vi "TDMS_set-motor-test.vi"() -> ()   [LabVIEW 2015]
uses:
  TDMS_use_state.ctl
  <vilib>/Platform/TimedLoop/XDataNode/timing_clust.ctl
  <vilib>/Platform/TimedLoop/XDataNode/nitl_modes.ctl
  <vilib>/Platform/TimedLoop/XDataNode/wakeup.ctl
  <vilib>/Rock Robotics/WPI/Utilities/WPI_GetSetVariantRefNum.vi
  <vilib>/platform/TimedLoop/XDataNode/XDataNode.xnode
  <vilib>/Platform/TimedLoop/XDataNode/XDNodeRunTimeDep.lvlib
panel:
  out "x != 0?":bool
  in  "New file?":bool
  in  "Run":bool
  in  "Start logging":bool
  in  "stop logging":bool
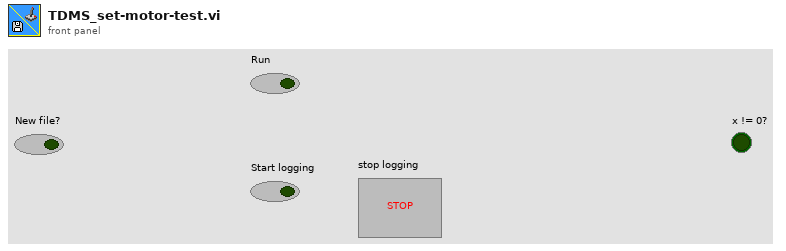
[diagram p1: front panel]
types:
  T1 = enum16{"open", "open or create", "create or replace", "create", "open (read-only)"}
  T2 = typedef "TDMS_use_state.ctl" = enum16{"Log", "Use", "Idle"}
  T3 = typedef "WPI_MotorControlDeviceRef.ctl" = cluster{"DeviceStatus":errorcluster, "Type":T4, "PWM":cluster{"PWM Channel":T5, "DeadBand":T6}, "CAN":cluster{"Device Number":u8, "Control Mode":T7, "Semaphore":T8, "Max Vout":dbl, "TalonSRX Control Mode":T9}, "Invert":bool}
  T4 = typedef "WPI_MotorControlType.ctl" = enum16{"PWM", "CAN", "CANTalonSRX"}
  T5 = typedef "FPGA_DIOPWMChannel.ctl" = enum8{"PWM 0", "PWM 1", "PWM 2", "PWM 3", "PWM 4", "PWM 5", "PWM 6", "PWM 7", "PWM 8", "PWM 9", "PWM MXP 0", "PWM MXP 1", "PWM MXP 2", "PWM MXP 3", "PWM MXP 4", "PWM MXP 5", "PWM MXP 6", "PWM MXP 7", "PWM MXP 8", "PWM MXP 9", "Invalid"}
  T6 = typedef "WPI_PWMDeadband.ctl" = cluster{"Name":string, "maxPositivePwm":i32, "minPositivePwm":i32, "centerPwm":i32, "maxNegativePwm":i32, "minNegativePwm":i32, "angularRange":u16}
  T7 = typedef "WPI_CANJaguar_ControlMode.ctl" = enum8{"Percent VBus", "Current", "Speed", "Position", "Voltage"}
  T8 = typedef "Semaphore RefNum" = refnum<k1>
  T9 = typedef "WPI_CANTalonSRX_APIControlMode.ctl" = enum8{"Percent VBus", "Speed", "Position", "Slave", "Unchanged / Invalid", "Voltage Compensation", "Current", "Motion Profile"}
  T10 = typedef "WPI_JoystickDevRef.ctl" = cluster{"Device":T11}
  T11 = typedef "WPI_JoystickDeviceEnum.ctl" = enum16{"USB 0", "USB 1", "USB 2", "USB 3", "USB 4", "USB 5"}
  T12 = typedef "XDNodeRunTimeDep.lvlib/timing_clust.ctl" = cluster{"Expected End [f-1]":u64, "Actual End [f-1]":u64, "Finished Late? [f-1]":bool, "Expected End [i-1]":u64, "Actual End [i-1]":u64, "Finished Late? [i-1]":bool, "Expected Start [i]":u64, "Actual Start [i]":u64, "Expected Start [f]":u64, "Actual Start [f]":u64, "Source Name":string, "Structure Name":string, "Period":i64, "Deadline":i64, "Offset":i64, "Start":i64, "Priority":i32, "Timeout":i32, "Mode":T13, "Wakeup Reason":T14, "Error":errorcluster, "Source Type":string, "Secondary Source Type":string, "Global End Time":u64, "Global Start Time":u64, "Frame Duration":u64, "Iteration Duration":u64, "Assigned CPU":i32, "I/O Scan Engine Mode":u32}
  T13 = typedef "XDNodeRunTimeDep.lvlib/nitl_modes.ctl" = enum32{"No Change", "Process missed periods, maintain original phase", "Discard missed periods, maintain original phase", "Process missed periods, ignore original phase", "Discard missed periods, ignore original phase"}
  T14 = typedef "XDNodeRunTimeDep.lvlib/wakeup.ctl" = enum32{"Normal", "Aborted", "Asynchronous wakeup", "Timing source error", "Timed loop error", "Timeout"}
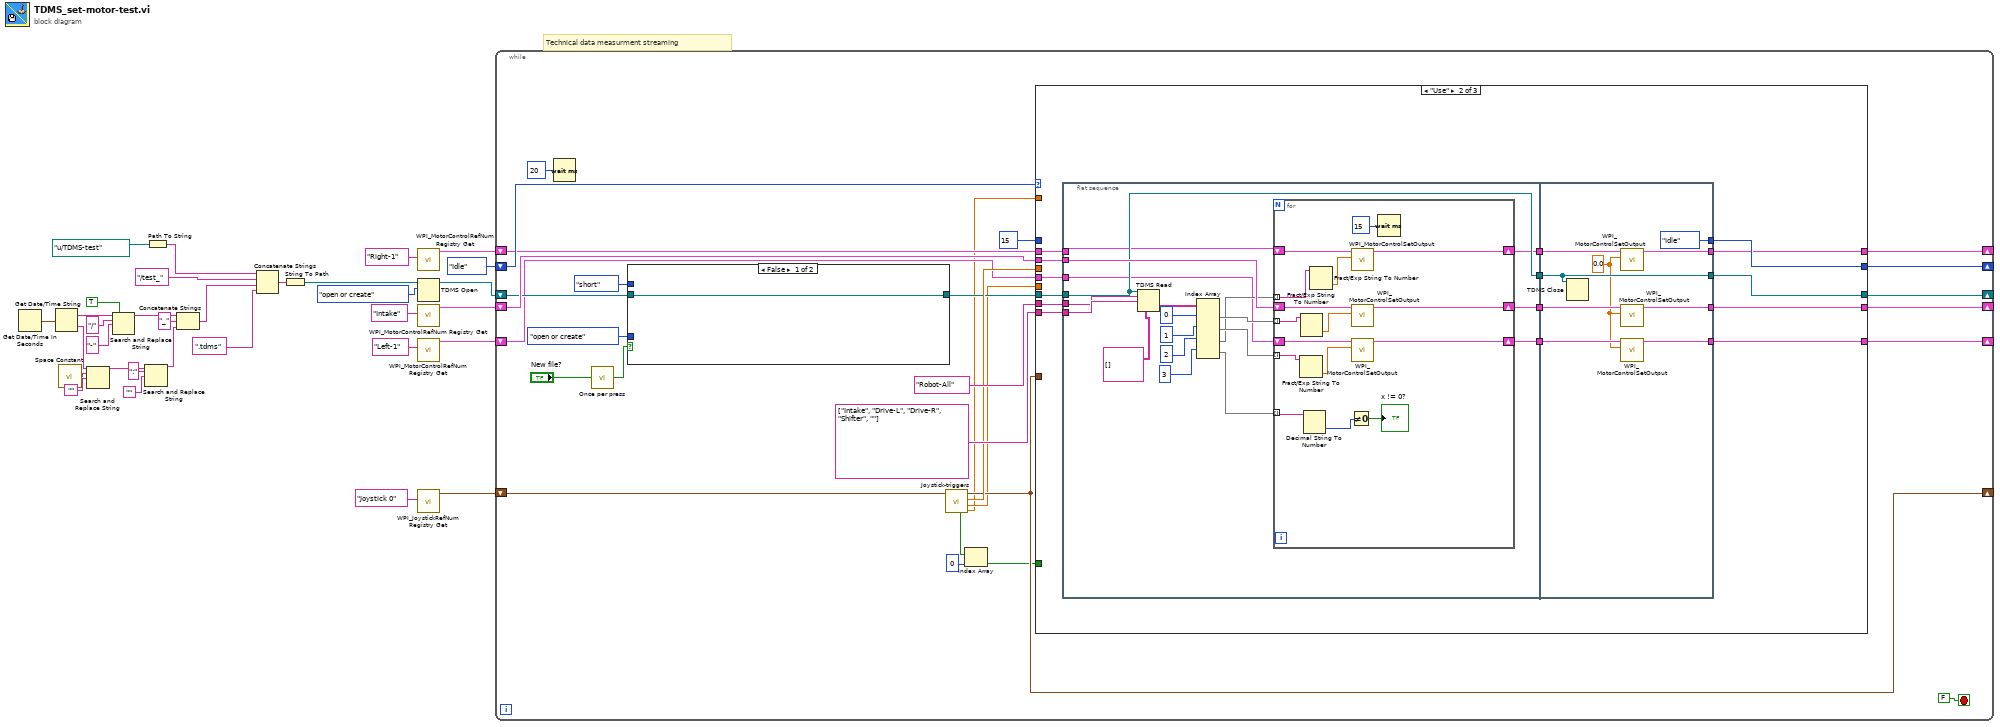
[diagram p0: block diagram]
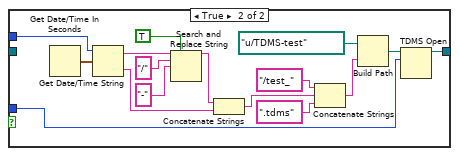
[diagram p2: hidden frame]
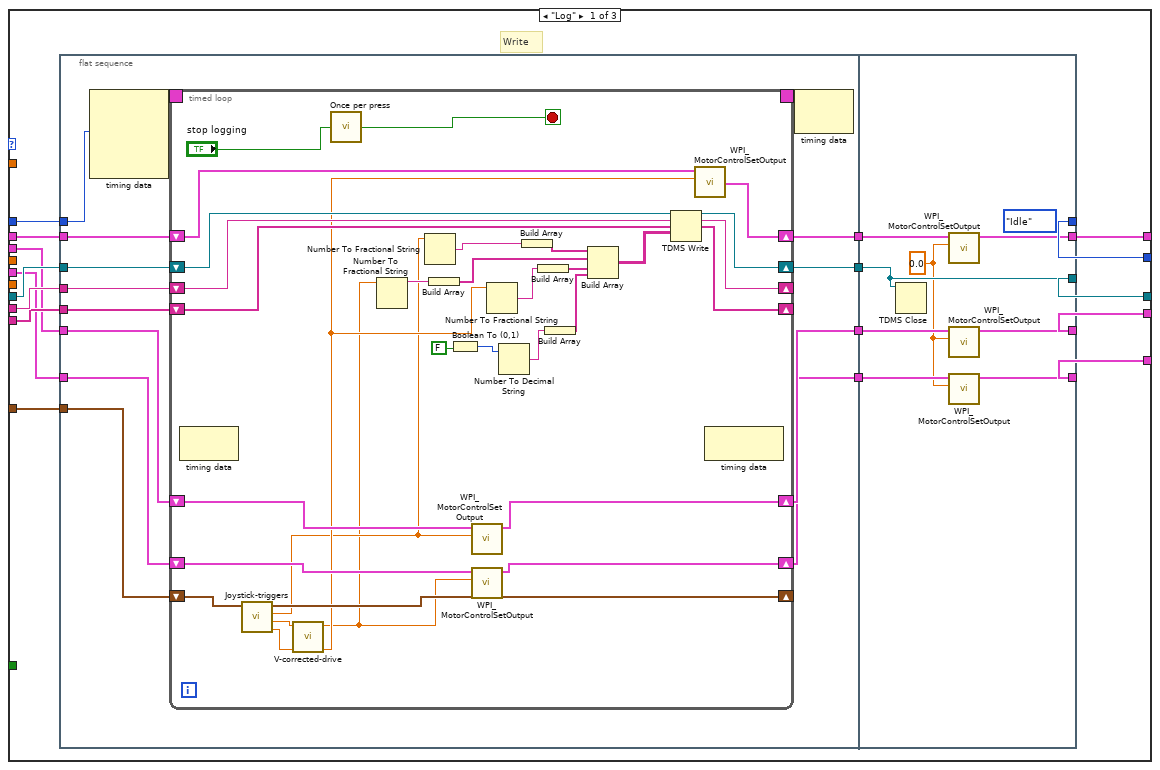
[diagram p3: hidden frame]
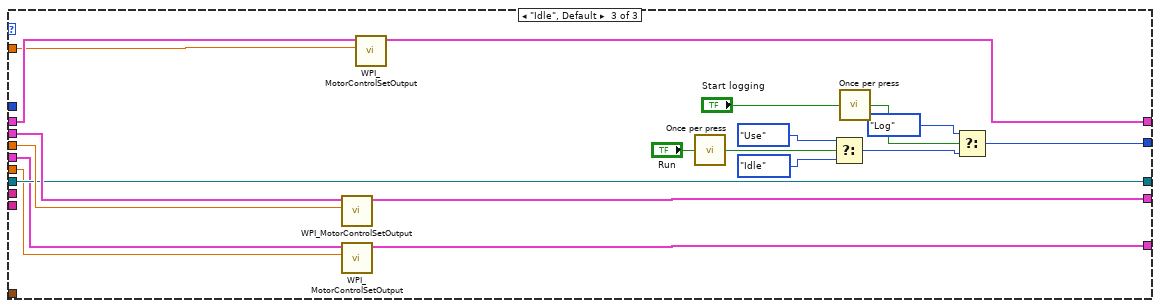
[diagram p4: hidden frame]
diagram:
  # "Technical data measurment streaming"
  n1 = Get Date/Time In Seconds() -> (seconds since 1Jan1904=w2:timestamp)
  n2 = Get Date/Time String(seconds (now)=w2) -> (date string=w16:string, time string=w13:string)  [unwired: 2 in]
  n3 = call <vilib>:"Space Constant.vi"() -> ("String"=w12:string)
  n4 = Search and Replace String(input string=w13, search string=w12, replace string="") -> (result string=w8:string)  [unwired: 5 in, 3 out]
  n5 = Search and Replace String(replace all?=TRUE ("replace all? (F)"), input string=w16, search string="/", replace string="-") -> (result string=w17:string)  [unwired: 4 in, 3 out]
  n6 = Search and Replace String(input string=w8, search string=":", replace string="") -> (result string=w5:string)  [unwired: 5 in, 3 out]
  n7 = Path To String(path=path "u:/TDMS-test" ("file path 3")) -> (string=w9:string)
  n8 = Concatenate Strings(w17, "_" ("string"), w5) -> (w21:string)
  n9 = Concatenate Strings(w9, "/test_" ("string"), w21, ".tdms" ("string")) -> (w14:string)
  n10 = String To Path(string=w14) -> (path=w1:path)
  n11 = call <vilib>:"WPI_MotorControlRefNum Registry Get.vi"("refnum name"="Right-1") -> ("MotorControlDevRef"=w24:T3)  [unwired: 9 in, 1 out]
  n12 = TDMS Open(10:T1."open or create" ("operation (0:open)"), 11:w1) -> (3:w27:refnum<k34>)  [unwired: 5 in, 1 out]
  n13 = call <vilib>:"WPI_MotorControlRefNum Registry Get.vi"("refnum name"="Intake") -> ("MotorControlDevRef"=w29:T3)  [unwired: 9 in, 1 out]
  n14 = call <vilib>:"WPI_MotorControlRefNum Registry Get.vi"("refnum name"="Left-1") -> ("MotorControlDevRef"=w25:T3)  [unwired: 9 in, 1 out]
  n15 = call <vilib>:"WPI_JoystickRefNum Registry Get.vi"("refnum name"="Joystick 0") -> ("JoystickDevRef"=w30:T10)  [unwired: 1 in, 9 out]
  n16 = while {
    shift-right: [w53] -> _
    shift-left: TDMS_use_state."Idle" ("Log or use?") -> [w54]
    shift-right: [w50] -> _
    shift-left: w30 -> [w51]
    shift-right: [w48] -> _
    shift-left: w29 -> [w49]
    shift-right: [w45] -> _
    shift-left: w27 -> [w43]
    shift-right: [w38] -> _
    shift-left: w25 -> [w40]
    shift-right: [w37] -> _
    shift-left: w24 -> [w39]
    stop <- FALSE stop-if-true
    n17 = Wait (ms)(milliseconds to wait=u32 20) -> ()  [unwired: 1 out]
    n18 = call "Once per press.vi"("In"="New file?") -> ("Out"=w47:bool)  [unwired: 2 in]
    n19 = case shown="False" w47 {
      tunnel: T1."open or create" ("operation (0:open)") -> [_ w76]
      tunnel: [w61 w77] -> w44
      tunnel: w43 -> [w61 _]
      tunnel: enum16{"short", "long", "abbreviated"}."short" ("date format (0)") -> [_ w63]
      frame False {
      }
      frame True {
        n20 = Get Date/Time In Seconds() -> (seconds since 1Jan1904=w69:timestamp)
        n21 = Get Date/Time String(date format (0)=w63, seconds (now)=w69) -> (date string=w65:string, time string=w71:string)  [unwired: 1 in]
        n22 = Search and Replace String(replace all?=TRUE ("replace all? (F)"), input string=w65, search string="/", replace string="-" ("replace string (\"\")")) -> (result string=w62:string)  [unwired: 4 in, 3 out]
        n23 = Concatenate Strings(w62, w71) -> (w70:string)
        n24 = Concatenate Strings("/test_", w70, ".tdms" ("name or relative path")) -> (w73:string)
        n25 = Build Path(base path=path "u:/TDMS-test" ("file path 3"), name or relative path=w73) -> (appended path=w68:path)
        n26 = TDMS Open(10:w76, 11:w68) -> (3:w77:refnum<k34>)  [unwired: 5 in, 1 out]
      }
    }
    n27 = call "Joystick-triggers.vi"("JoystickDevRef"=w51) -> ("Right out"=w35:dbl, "Left out"=w36:dbl, "x+y"=w52:dbl, "JoystickDevRef out"=w50:T10, "Buttons"=w42:bool[])  [unwired: 6 in]
    n28 = Index Array(array=w42, index=0) -> (element=w33:bool)
    n29 = case shown="\"Use\"" w54 {
      tunnel: w44 -> [w92 w167 w221]
      tunnel: "Robot-All" ("group name in (Untitled)") -> [w91 w168 _]
      tunnel: string[] ["Intake", "Drive-L", "Drive-R", "Shifter", ""] ("channel name(s) in (Untitled)") -> [w90 w169 _]
      tunnel: w49 -> [w89 w170 w233]
      tunnel: i64 15 ("Log rate") -> [w88 _ _]
      tunnel: w52 -> [_ _ w232]
      tunnel: [w87 w164 w227] -> w53
      tunnel: w50 -> [w86 _ _]
      tunnel: [w85 w163 w226] -> w48
      tunnel: [w84 w162 w221] -> w45
      tunnel: w40 -> [w83 w161 w220]
      tunnel: w39 -> [w82 w160 w219]
      tunnel: [w79 w157 w218] -> w38
      tunnel: [w78 w156 w217] -> w37
      tunnel: w36 -> [_ _ w216]
      tunnel: w35 -> [_ _ w215]
      tunnel: w33 -> [_ _ _]
      frame "Log" {
        # "Write"
        n30 = flat-sequence {
          tunnel: w92 -> [w108]
          tunnel: w91 -> [w107]
          tunnel: w90 -> [w106]
          tunnel: w89 -> [w103]
          tunnel: [w102] -> w94
          tunnel: [w101] -> w93
          tunnel: w88 -> [w100]
          tunnel: w86 -> [w99]
          tunnel: w83 -> [w98]
          tunnel: w82 -> [w97]
          tunnel: [w96] -> w81
          tunnel: [w95] -> w80
          tunnel: w94 -> [w155]
          tunnel: w93 -> [w152]
          tunnel: [TDMS_use_state."Idle" ("Log or use?")] -> w87
          tunnel: [w153] -> w85
          tunnel: [w152] -> w84
          tunnel: w81 -> [w151]
          tunnel: w80 -> [w150]
          tunnel: [w148] -> w79
          tunnel: [w147] -> w78
          frame #0 {
            n31 = node-c288(w100) -> (w105:T12)  [unwired: 3 in]
            n32 = timed-loop {
              timing: w105 -> [_]
              timing-out: [_] -> w104
              shift-right: [w135] -> _
              shift-left: w107 -> [w139]
              shift-right: [w118] -> _
              shift-left: w106 -> [w123]
              shift-right: [w136] -> w101
              shift-left: w108 -> [w140]
              shift-right: [w137] -> w102
              shift-left: w103 -> [w138]
              shift-right: [w133] -> _
              shift-left: w99 -> [w134]
              shift-right: [w128] -> w96
              shift-left: w98 -> [w130]
              shift-right: [w127] -> w95
              shift-left: w97 -> [w129]
              stop <- w131 stop-if-true
              n33 = node-c288() -> ()  [unwired: 1 in, 1 out]
              n34 = call "Joystick-triggers.vi"("JoystickDevRef"=w134) -> ("Right out"=w125:dbl, "Left out"=w126:dbl, "x+y"=w114:dbl, "JoystickDevRef out"=w133:T10)  [unwired: 6 in, 1 out]
              n35 = call "V-corrected-drive.vi"("R-IN"=w125, "L-IN 2"=w126) -> ("Right out"=w115:dbl, "Left out"=w113:dbl)  [unwired: 8 in]
              n36 = call "Once per press.vi"("In"="stop logging") -> ("Out"=w131:bool)  [unwired: 2 in]
              n37 = Number To Fractional String(number=w113) -> (F-format string=w120:string)  [unwired: 3 in]
              n38 = Number To Fractional String(number=w114) -> (F-format string=w124:string)  [unwired: 3 in]
              n39 = Build Array(w120) -> (w119:string[])
              n40 = Boolean To (0,1)(Boolean=FALSE) -> (0, 1=w111:i16)
              n41 = call <vilib>:"WPI_MotorControlSetOutput.vi"("Output"=w114, "MotorControlDevRef"=w138) -> ("MotorControlDevRef"=w137:T3)  [unwired: 7 in, 2 out]
              n42 = call <vilib>:"WPI_MotorControlSetOutput.vi"("Output"=w113, "MotorControlDevRef"=w130) -> ("MotorControlDevRef"=w128:T3)  [unwired: 7 in, 2 out]
              n43 = Number To Fractional String(number=w115) -> (F-format string=w117:string)  [unwired: 3 in]
              n44 = Number To Decimal String(number=w111) -> (decimal integer string=w110:string)  [unwired: 1 in]
              n45 = Build Array(w124) -> (w121:string[])
              n46 = Build Array(w117) -> (w116:string[])
              n47 = Build Array(w110) -> (w109:string[])
              n48 = Build Array(w121, w119, w116, w109) -> (w122:string[][])
              n49 = TDMS Write(0:w140, 5:w139, 7:w123, 9:w122) -> (4:w136:refnum<k34>, 6:w135:string, 8:w118:string[])  [unwired: 2 in, 1 out]
              n50 = call <vilib>:"WPI_MotorControlSetOutput.vi"("Output"=w115, "MotorControlDevRef"=w129) -> ("MotorControlDevRef"=w127:T3)  [unwired: 7 in, 2 out]
              n51 = node-c288() -> ()  [unwired: 1 in, 1 out]
            }
            n52 = node-c288(w104) -> ()  [unwired: 1 out]
          }
          frame #1 {
            w149 = 0.0 ("Output")
            n53 = TDMS Close(11:w152) -> ()  [unwired: 1 in, 2 out]
            n54 = call <vilib>:"WPI_MotorControlSetOutput.vi"("Output"=w149, "MotorControlDevRef"=w150) -> ("MotorControlDevRef"=w147:T3)  [unwired: 7 in, 2 out]
            n55 = call <vilib>:"WPI_MotorControlSetOutput.vi"("Output"=w149, "MotorControlDevRef"=w155) -> ("MotorControlDevRef"=w153:T3)  [unwired: 7 in, 2 out]
            n56 = call <vilib>:"WPI_MotorControlSetOutput.vi"("Output"=w149, "MotorControlDevRef"=w151) -> ("MotorControlDevRef"=w148:T3)  [unwired: 7 in, 2 out]
          }
        }
      }
      frame "Use" {
        n57 = flat-sequence {
          tunnel: w170 -> [w186]
          tunnel: w169 -> [w185]
          tunnel: w168 -> [w184]
          tunnel: w167 -> [w183]
          tunnel: [w183] -> w166
          tunnel: [w182] -> w165
          tunnel: w161 -> [w177]
          tunnel: w160 -> [w176]
          tunnel: [w175] -> w159
          tunnel: [w174] -> w158
          tunnel: w166 -> [w211]
          tunnel: w165 -> [w214]
          tunnel: [TDMS_use_state."Idle" ("Log or use?")] -> w164
          tunnel: [w212] -> w163
          tunnel: [w211] -> w162
          tunnel: w159 -> [w210]
          tunnel: w158 -> [w209]
          tunnel: [w208] -> w157
          tunnel: [w207] -> w156
          frame #0 {
            n58 = TDMS Read(0:w183, 5:w184, 7:w185, 12:string[][] [] ("appended array")) -> (10:w188:string[][])  [unwired: 4 in, 5 out]
            n59 = Index Array(array=w188, index (row) #1=0 ("index (row)"), index (row) #2=1 ("index (row)"), index (row) #3=2 ("index (row)"), index (row) #4=3 ("index (row)")) -> (element #1=w187:string[], element #2=w179:string[], element #3=w178:string[], element #4=w171:string[])  [unwired: 4 in]
            n60 = for {
              tunnel: w187 -> [w196] mode=indexing
              shift-right: [w204] -> w182
              shift-left: w186 -> [w205]
              tunnel: w179 -> [w194] mode=indexing
              tunnel: w178 -> [w197] mode=indexing
              shift-right: [w200] -> w175
              shift-left: w177 -> [w202]
              shift-right: [w199] -> w174
              shift-left: w176 -> [w201]
              tunnel: w171 -> [w192] mode=indexing
              n61 = Fract/Exp String To Number(string=w194) -> (number=w193:dbl)  [unwired: 3 in, 1 out]
              n62 = Fract/Exp String To Number(string=w196) -> (number=w195:dbl)  [unwired: 3 in, 1 out]
              n63 = Decimal String To Number(string=w192) -> (number=w191:i32)  [unwired: 2 in, 1 out]
              n64 = Fract/Exp String To Number(string=w197) -> (number=w198:dbl)  [unwired: 3 in, 1 out]
              n65 = Not Equal To 0?(x=w191) -> (x != 0?=→"x != 0?":bool)
              n66 = call <vilib>:"WPI_MotorControlSetOutput.vi"("Output"=w198, "MotorControlDevRef"=w201) -> ("MotorControlDevRef"=w199:T3)  [unwired: 7 in, 2 out]
              n67 = call <vilib>:"WPI_MotorControlSetOutput.vi"("Output"=w195, "MotorControlDevRef"=w205) -> ("MotorControlDevRef"=w204:T3)  [unwired: 7 in, 2 out]
              n68 = call <vilib>:"WPI_MotorControlSetOutput.vi"("Output"=w193, "MotorControlDevRef"=w202) -> ("MotorControlDevRef"=w200:T3)  [unwired: 7 in, 2 out]
              n69 = Wait (ms)(milliseconds to wait=u32 15) -> ()  [unwired: 1 out]
            }
          }
          frame #1 {
            w206 = 0.0 ("Output")
            n70 = TDMS Close(11:w211) -> ()  [unwired: 1 in, 2 out]
            n71 = call <vilib>:"WPI_MotorControlSetOutput.vi"("Output"=w206, "MotorControlDevRef"=w209) -> ("MotorControlDevRef"=w207:T3)  [unwired: 7 in, 2 out]
            n72 = call <vilib>:"WPI_MotorControlSetOutput.vi"("Output"=w206, "MotorControlDevRef"=w214) -> ("MotorControlDevRef"=w212:T3)  [unwired: 7 in, 2 out]
            n73 = call <vilib>:"WPI_MotorControlSetOutput.vi"("Output"=w206, "MotorControlDevRef"=w210) -> ("MotorControlDevRef"=w208:T3)  [unwired: 7 in, 2 out]
          }
        }
      }
      frame "Idle", Default {
        n74 = call <vilib>:"WPI_MotorControlSetOutput.vi"("Output"=w232, "MotorControlDevRef"=w233) -> ("MotorControlDevRef"=w226:T3)  [unwired: 7 in, 2 out]
        n75 = call <vilib>:"WPI_MotorControlSetOutput.vi"("Output"=w216, "MotorControlDevRef"=w220) -> ("MotorControlDevRef"=w218:T3)  [unwired: 7 in, 2 out]
        n76 = call <vilib>:"WPI_MotorControlSetOutput.vi"("Output"=w215, "MotorControlDevRef"=w219) -> ("MotorControlDevRef"=w217:T3)  [unwired: 7 in, 2 out]
        n77 = call "Once per press.vi"("In"="Run") -> ("Out"=w222:bool)  [unwired: 2 in]
        n78 = Select(t=TDMS_use_state."Use" ("Log or use?"), s=w222, f=TDMS_use_state."Idle") -> (s? t:f=w231:T2)
        n79 = call "Once per press.vi"("In"="Start logging") -> ("Out"=w224:bool)  [unwired: 2 in]
        n80 = Select(t=TDMS_use_state."Log" ("Log or use?"), s=w224, f=w231) -> (s? t:f=w227:T2)
      }
    }
  }
